vi "From JSON.vi"(7 "LVClass Serializer":refnum<class "JSONtext LVClass Serializer.lvclass">, 8 "error in (no error)":errorcluster, 10 "<JSON>":string, 11 "Mock JSON Serializable in":refnum<class "Mock JSON Serializable.lvclass">) -> (0 "error out":errorcluster, 3 "Mock JSON Serializable out":refnum<class "Mock JSON Serializable.lvclass">)   [LabVIEW 2017, in "JSON Serializable Serializer Tests.lvlib" / "Mock JSON Serializable.lvclass"]
doc: "Reads data from a JSON string."
uses:
  Mock JSON Serializable.lvclass
  <vilib>/JDP Science/JSONtext/LVClass Serializer/JSONtext LVClass Serializer.lvclass
  Mock JSON Serializable.lvclass/Mock JSON Serializable.ctl
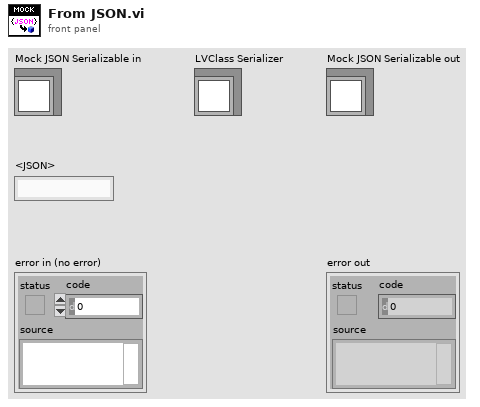
[diagram p1: front panel]
types:
  T1 = cluster{"LVClass Serializer":refnum<class "JSONtext LVClass Serializer.lvclass">, "<JSON>":string, "error in (no error)":errorcluster}
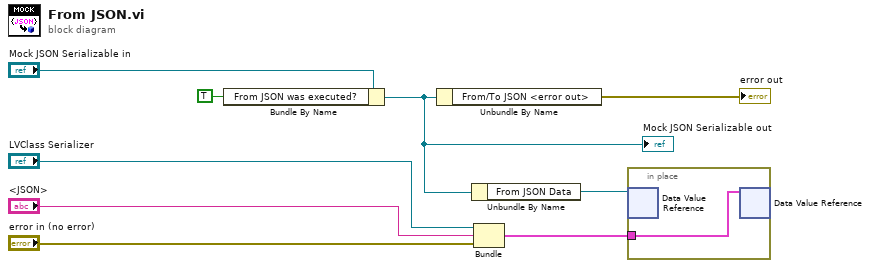
[diagram p0: block diagram]
diagram:
  n1 = Bundle By Name(cluster="Mock JSON Serializable in", "From JSON was executed?"=TRUE) -> (w2:refnum<class "Mock JSON Serializable.lvclass">)
  "Mock JSON Serializable out" <- w2
  n2 = Unbundle By Name(w2) -> ("From/To JSON <error out>"=→"error out":errorcluster)
  n3 = Unbundle By Name(w2) -> ("From JSON Data"=w7:refnum<data-value>)
  n4 = Bundle("LVClass Serializer"="LVClass Serializer", "<JSON>"="<JSON>", "error in (no error)"="error in (no error)") -> (w6:T1)  [unwired: 1 in]
  n5 = in-place {
    in-place-border: w6 -> [w10]
    n6 = in-place-dvr #1(w7) -> ()  [unwired: 2 out]
    n7 = in-place-dvr #1(w10) -> ()  [unwired: 2 out]
  }
